vi "TagBus_Get Tag Keys (DVR).vi"(10 "Tag Key Array":string[](array[string])=["EnergyStorage_kW"], 11 "TagBus DVR":refnum<data-value>) -> (2 "Index Array":i32[](array[numeric]), 3 "TagBus DVR out":refnum<data-value>)   [LabVIEW 2015, in "TagBus.lvclass"]
uses:
  TagBus.lvclass
  TagBus.lvclass/TagBus.ctl
  <vilib>/NI/Tag Bus/dictionary/locate tag of unknown type.vi
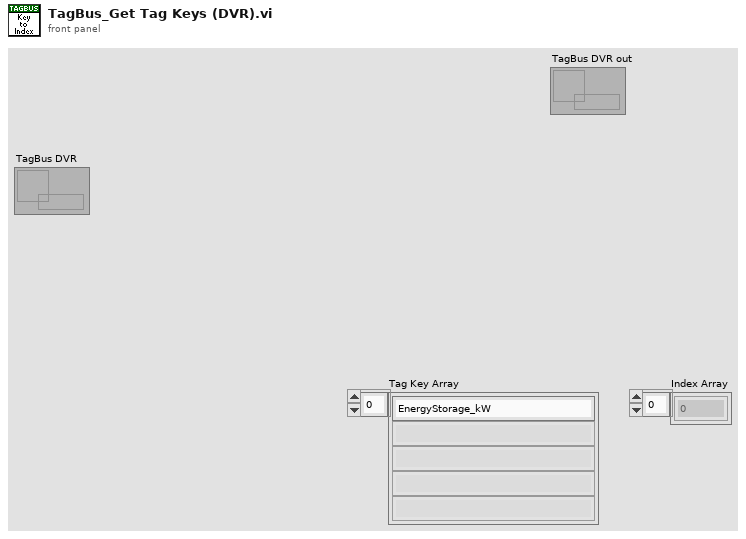
[diagram p1: front panel]
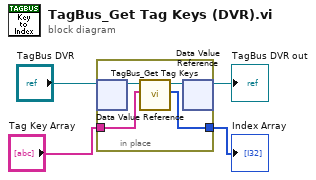
[diagram p0: block diagram]
diagram:
  n1 = in-place {
    in-place-border: "Tag Key Array" -> [w6]
    in-place-border: [w5] -> w4
    n2 = in-place-dvr #1("TagBus DVR") -> (w8:refnum<class "TagBus.lvclass">)  [unwired: 1 out]
    n3 = call "TagBus_Get Tag Keys.vi"("Tag Keys"=w6, "TagBus"=w8) -> ("Index Array"=w5:i32[], "TagBus out"=w7:refnum<class "TagBus.lvclass">)  [unwired: 8 in]
    n4 = in-place-dvr #1(w7) -> (→"TagBus DVR out":refnum<data-value>)  [unwired: 1 out]
  }
  "Index Array" <- w4
